vi "update config.vi"(8 "error in (no error)":errorcluster, 10 "user configurations":T2={"vst_device"=["VST_1", "VST_2"], "RF gain "=10.0, "buffer size"=524288, "center frequency (Hz) "=1000000000.0, "P2P sample rate"=200000000.0, "mode"=enum."5785 - 2*180MHz", "devicess"=["IF_transiver_0", "IF_transiver_1", "IF_transiver_2"], "file paths"=[path "C:/Users/PXIe8108_Demo/Documents/CHAIM DATA/chaim/5785_sync_for_elbit/data/pdw_test_file.tdms", path "C:/Users/PXIe8108_Demo/Documents/CHAIM DATA/chaim/5785_sync_for_elbit/data/pdw_test_file_1.tdms", path "C:/Users/PXIe8108_Demo/Documents/CHAIM DATA/chaim/5785_sync_for_elbit/data/pdw_test_file_2.tdms", path "C:/Users/PXIe8108_Demo/Documents/CHAIM DATA/chaim/5785_sync_for_elbit/data/pdw_test_file_3.tdms", path "C:/Users/PXIe8108_Demo/Documents/CHAIM DATA/chaim/5785_sync_for_elbit/data/pdw_test_file_4.tdms"], "gen for df"=FALSE}, 11 "pulse_gen_and_detect_p2p in":refnum<class "pulse_gen_and_detect_p2p.lvclass">) -> (0 "error out":errorcluster, 1 "min frequency":dbl, 2 "max frequency":dbl, 3 "pulse_gen_and_detect_p2p out":refnum<class "pulse_gen_and_detect_p2p.lvclass">)   [LabVIEW 2021, in "pulse_gen_and_detect_p2p.lvclass"]
uses:
  pulse_gen_and_detect_p2p.lvclass
  <vilib>/userdefined/High Color/nirio_resource_hc.ctl
  pulse_gen_and_detect_p2p.lvclass/pulse_gen_and_detect_p2p.ctl
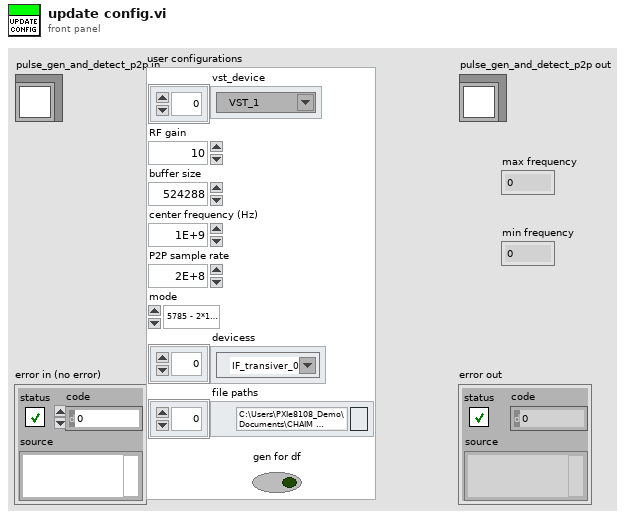
[diagram p1: front panel]
types:
  T1 = typedef "nirio_resource_hc.ctl" = tag
  T2 = cluster{"vst_device":refnum<k15>[], "RF gain ":dbl, "buffer size":u32, "center frequency (Hz) ":dbl, "P2P sample rate":dbl, "mode":enum16{"USRP - 180MHz", "5785 - 2*180MHz", "5785 - 3.2GHz", "P2P - VST"}, "devicess":T1[], "file paths":path[], "gen for df":bool}
  T3 = cluster{"min PW (fft cycels)":u16, "max PW (fft cycels)":u16, "max gap (fft cycels)":u8, "detection bar (liniar amp)":fxp<+,64,63>, "peak detect":bool}
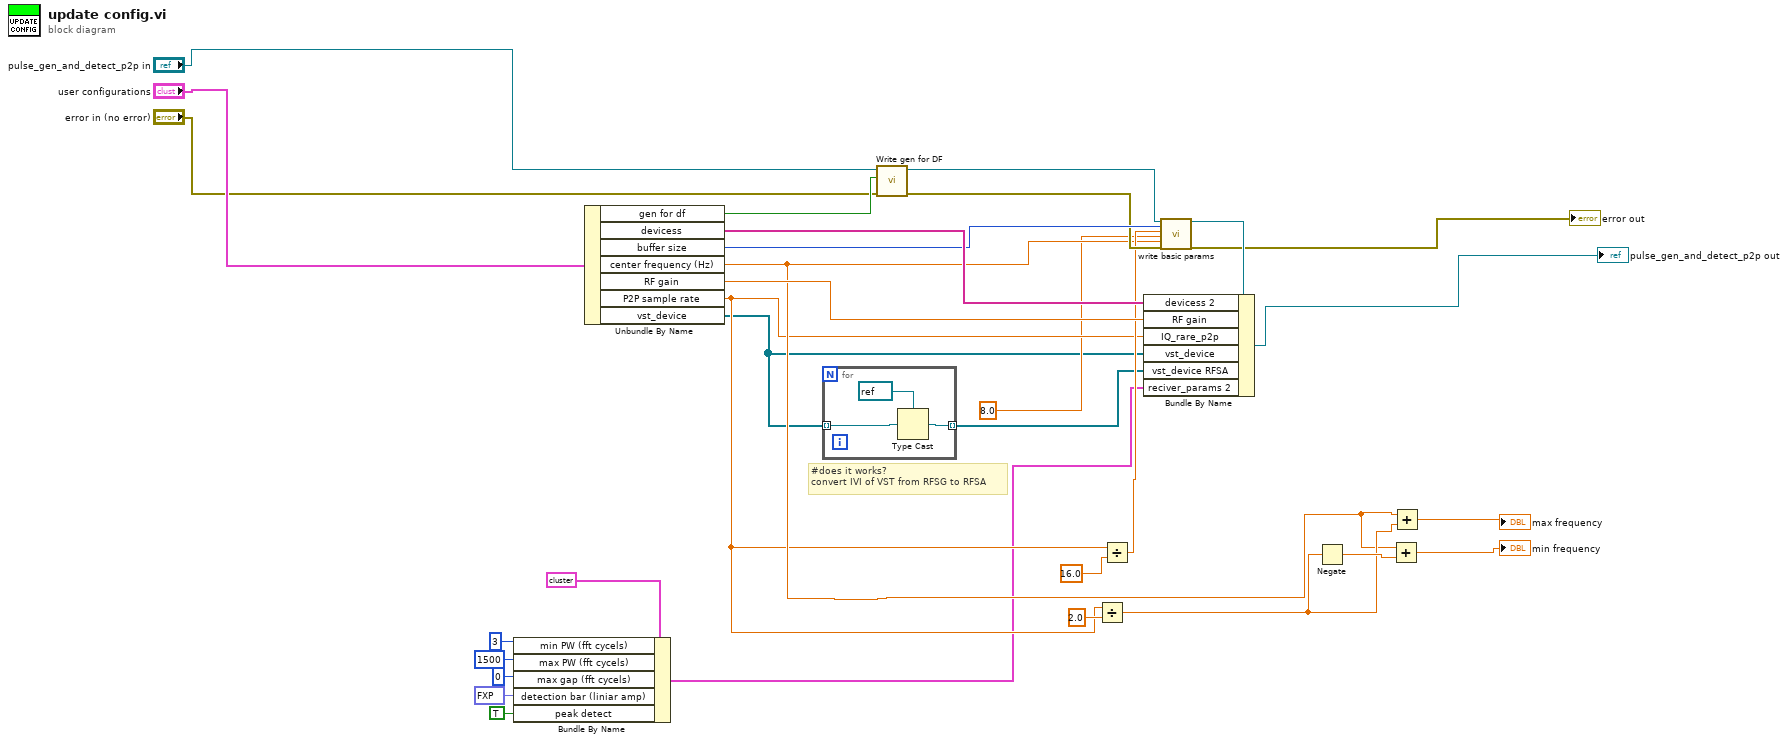
[diagram p0: block diagram]
diagram:
  # "#does it works?\nconvert IVI of VST from RFSG to RFSA"
  n1 = Bundle By Name(cluster=T3 {"min PW (fft cycels)"=0, "max PW (fft cycels)"=0, "max gap (fft cycels)"=0, "detection bar (liniar amp)"=0.0, "peak detect"=FALSE} ("reciver_params 2"), "min PW (fft cycels)"=u16 3, "max PW (fft cycels)"=u16 1500, "max gap (fft cycels)"=u8 0, "detection bar (liniar amp)"=fxp<+,64,63> 5000.0, "peak detect"=TRUE) -> (w6:T3)
  n2 = Unbundle By Name("user configurations") -> ("gen for df"=w27:bool, "devicess"=w31:T1[], "buffer size"=w30:u32, "center frequency (Hz)"=w19:dbl, "RF gain"=w25:dbl, "P2P sample rate"=w18:dbl, "vst_device"=w9:refnum<k15>[])
  n3 = for {
    tunnel: w9 -> [w34] mode=indexing
    tunnel: [w33] -> w8 mode=indexing
    n4 = Type Cast(type=refnum<k15> refnum ("resource name"), x=w34) -> (*(type *) &x=w33:refnum<k15>)
  }
  n5 = call-dynamic "Write gen for DF.vi"("error in (no error)"="error in (no error)", "gen for DF"=w27, "device_type in"="pulse_gen_and_detect_p2p in") -> ("error out"=w26:errorcluster, "device_type out"=w28:refnum<class "pulse_gen_and_detect_p2p.lvclass">)  [unwired: 7 in]
  n6 = Divide(x=w18, y=2.0) -> (x/y=w23:dbl)
  n7 = Divide(x=w18, y=16.0 ("Fs  FPGA")) -> (x/y=w20:dbl)
  n8 = call-dynamic "write basic params.vi"("device_type in"=w28, "buffer size"=w30, "Fs  FPGA"=w20, "SPC"=8.0 ("t"), "center frequency (Hz)"=w19, "error in (no error)"=w26) -> ("device_type out"=w29:refnum<class "pulse_gen_and_detect_p2p.lvclass">, "error out"=→"error out":errorcluster)  [unwired: 12 in]
  n9 = Bundle By Name(cluster=w29, "devicess 2"=w31, "RF gain"=w25, "IQ_rare_p2p"=w18, "vst_device"=w9, "vst_device RFSA"=w8, "reciver_params 2"=w6) -> (→"pulse_gen_and_detect_p2p out":refnum<class "pulse_gen_and_detect_p2p.lvclass">)
  n10 = Negate(x=w23) -> (-x=w24:dbl)
  n11 = Add(x=w19, y=w24) -> (x+y=→"min frequency":dbl)
  n12 = Add(x=w19, y=w23) -> (x+y=→"max frequency":dbl)
